vi "Do.vi"(8 "error in (no error)":errorcluster, 10 "Actor in":refnum<class "Actor.lvclass">, 11 "Verify and Check-in Msg":refnum<class "Verify and Check-in Msg.lvclass">) -> (0 "error out":errorcluster, 2 "Actor out":refnum<class "Actor.lvclass">)   [LabVIEW 2023, in "Incoming Rooms Manager Model Interface.lvlib" / "Verify and Check-in Msg.lvclass"]
doc: "This VI delivers the message to the actor by calling the appropriate method(s) on the actor."
uses:
  Verify and Check-in Msg.lvclass
  Verify and Check-in Msg.lvclass/Verify and Check-in Msg.ctl
  9ef47adc-f318-494c-9b8b-6df3216d6863.vi
  Rooms Manager Model/Incoming Rooms Manager Model Interface.lvclass
  <vilib>/ActorFramework/Actor/Actor.lvclass
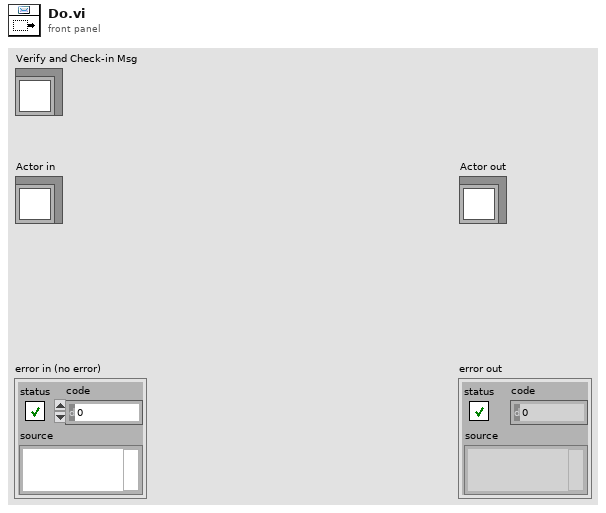
[diagram p1: front panel]
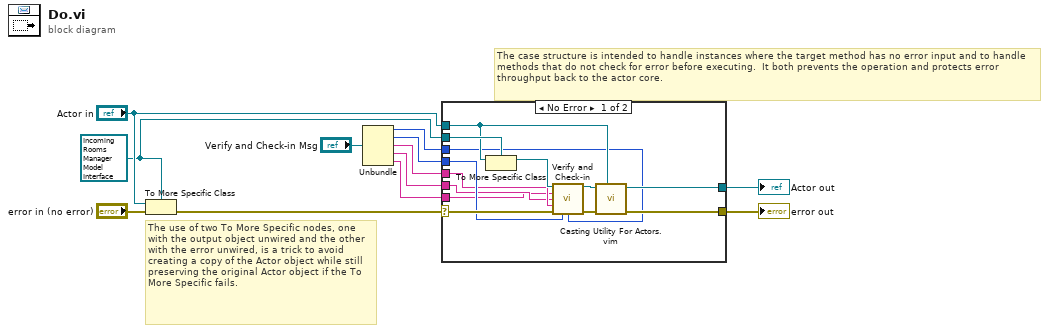
[diagram p0: block diagram]
diagram:
  w6 = refnum<class "Incoming Rooms Manager Model Interface.lvclass"> refnum ("Actor in")
  # "The use of two To More Specific nodes, one with the output object unwired and the other with the error unwired, is a trick to avoid creating a copy of the Actor object while still preserving the original Actor object if the To More Specific fails."
  # "The case structure is intended to handle instances where the target method has no error input and to handle methods that do not check for error before executing.  It both prevents the operation and protects error throughput back to the actor core."
  n1 = To More Specific Class(target class=w6, reference="Actor in", error in="error in (no error)") -> (error out=w10:errorcluster)  [unwired: 1 out]
  n2 = Unbundle("Verify and Check-in Msg") -> (w5:u32, w4:u32, w3:string, w2:string, w1:string)
  n3 = case shown="No Error" w10 {
    selector: w10 -> [w25 w27]
    tunnel: [w19 w27] -> w9
    tunnel: [w20 w26] -> w8
    tunnel: "Actor in" -> [w22 w26]
    tunnel: w6 -> [w23 _]
    tunnel: w5 -> [w17 _]
    tunnel: w4 -> [w16 _]
    tunnel: w3 -> [w15 _]
    tunnel: w2 -> [w14 _]
    tunnel: w1 -> [w13 _]
    frame No Error {
      n4 = To More Specific Class(target class=w23, reference=w22) -> (specific class reference=w24:refnum<class "Incoming Rooms Manager Model Interface.lvclass">)  [unwired: 1 in, 1 out]
      n5 = call-dynamic "Verify and Check-in.vi"("Incoming Rooms Manager Model Interface in"=w24, "Room No"=w13, "Guest Contact Number"=w14, "Primary Guest Name"=w15, "error in (no error)"=w25, "Adults"=w16, "Children"=w17) -> ("Incoming Rooms Manager Model Interface out"=w21:refnum<class "Incoming Rooms Manager Model Interface.lvclass">, "error out"=w18:errorcluster)  [unwired: 7 in]
      n6 = call "Casting Utility For Actors.vim"("type"=w22, "error in (no error)"=w18, "Actor in"=w21) -> ("error out"=w19:errorcluster, "Actor out"=w20:refnum<class "Actor.lvclass">)  [unwired: 7 in]
    }
    frame Error {
      # "If type check fails, pass the original object out again."
    }
  }
  "error out" <- w9
  "Actor out" <- w8
